vi "Cylindrical E-Field Meter.vi"() -> ()   [LabVIEW 2012]
panel:
  out "x/y":dbl
  out "ADC Reading":i64
  out "Voltage on Op Amp output":dbl
  in  "Buffering size":i32=100
  out "Continuous Measurements":dbl[](graph)
  out "N of Iterations":i32
  in  "Buffering size":i32=100
  in  "stop":bool
  in  "Ey Field (V)":dbl(knob) scale=-16000.0..16000.0
  in  "Ex Field (V)":dbl(knob) scale=-1000.0..1000.0
  out "Measurements taken every 2*Pi":dbl[](graph)
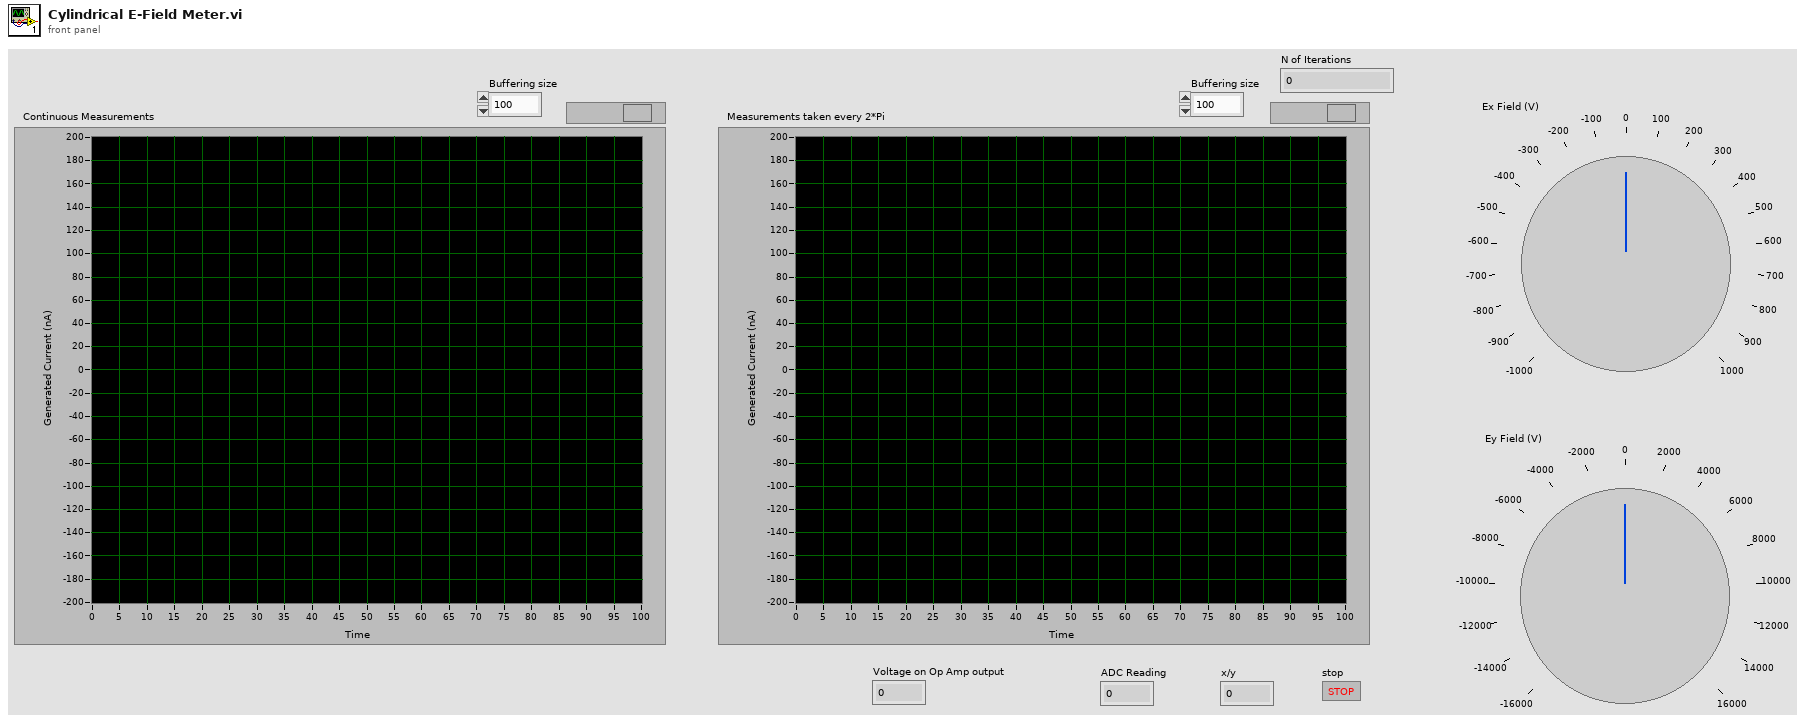
[diagram p1: front panel]
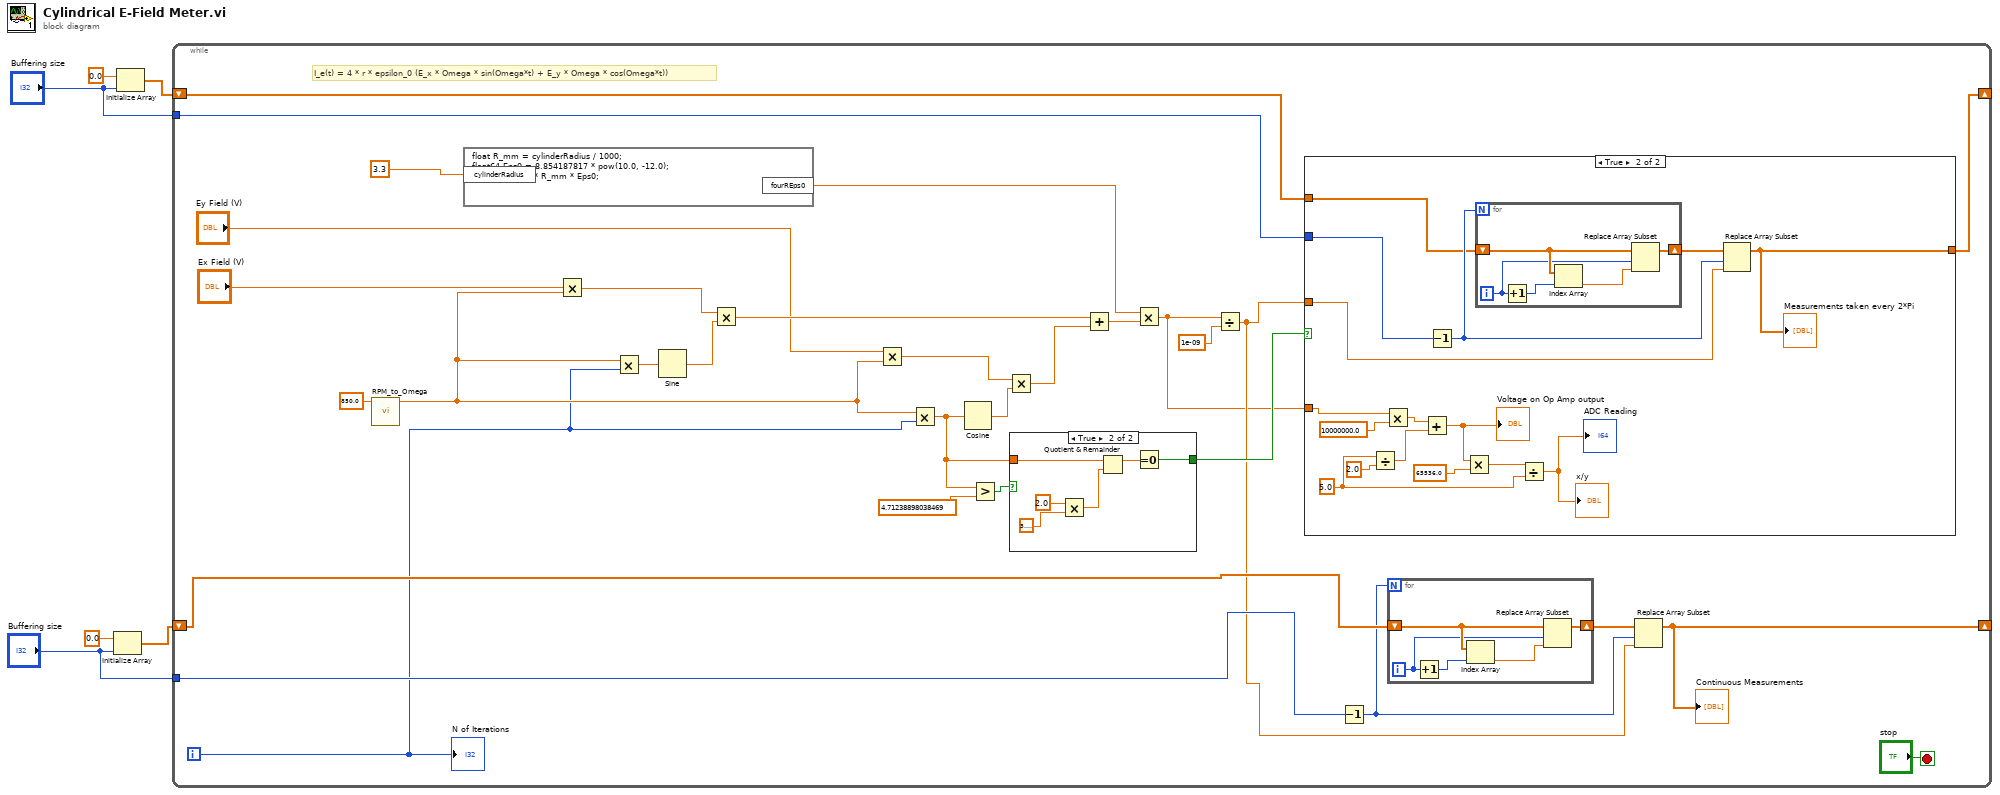
[diagram p0: block diagram]
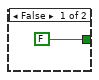
[diagram p2: hidden frame]
diagram:
  n1 = Initialize Array(0.0 ("element"), "Buffering size") -> (w3:dbl[])
  n2 = Initialize Array(0.0 ("element"), "Buffering size") -> (w5:dbl[])
  n3 = while {
    tunnel: "Buffering size" -> [w36]
    shift-right: [w34] -> _
    shift-left: w5 -> [w35]
    shift-right: [w12] -> _
    shift-left: w3 -> [w21]
    tunnel: "Buffering size" -> [w20]
    i -> [w9]
    stop <- "stop" stop-if-true
    # "I_e(t) = 4 * r * epsilon_0 (E_x * Omega * sin(Omega*t) + E_y * Omega * cos(Omega*t))"
    n4 = call "RPM_to_Omega.vi"("Rotational Speed (RPM)"=850.0) -> ("Angular Velocity (omega)"=w23:dbl)  [unwired: 10 in]
    n5 = formula code="float R_mm = cylinderRadius / 1000;\nfloat64 Eps0 = 8.854187817 * pow(10.0, -12.0);\nfourREps0 = 4 * R_mm * Eps0;"("cylinderRadius"=3.3 ("input variable")) -> ("fourREps0"=w10:dbl)
    n6 = Multiply(x="Ex Field (V)", y=w23) -> (x*y=w33:dbl)
    n7 = Multiply(x=w23, y=w9) -> (x*y=w18:dbl)
    n8 = Sine(x=w18) -> (sin(x)=w31:dbl)
    n9 = Multiply(x=w33, y=w31) -> (x*y=w29:dbl)
    n10 = Multiply(x="Ey Field (V)", y=w23) -> (x*y=w32:dbl)
    n11 = Multiply(x=w23, y=w9) -> (x*y=w16:dbl)
    n12 = Cosine(x=w16) -> (cos(x)=w30:dbl)
    n13 = Greater?(x=w16, y=4.71238898038469) -> (0:w15:bool)
    n14 = Multiply(x=w32, y=w30) -> (x*y=w28:dbl)
    n15 = case shown="True" w15 {
      tunnel: [FALSE w48] -> w22
      tunnel: w16 -> [_ w44]
      frame False {
      }
      frame True {
        n16 = Multiply(x=2.0, y=3.141592653589793) -> (x*y=w45:dbl)
        n17 = Quotient & Remainder(x=w44, y=w45) -> (x-y*floor(x/y)=w49:dbl)  [unwired: 1 out]
        n18 = Equal To 0?(x=w49) -> (x = 0?=w48:bool)
      }
    }
    n19 = Add(x=w29, y=w28) -> (x+y=w27:dbl)
    n20 = Multiply(x=w10, y=w27) -> (x*y=w11:dbl)
    n21 = Divide(x=w11, y=1e-09) -> (x/y=w19:dbl)
    n22 = case shown="True" w22 {
      tunnel: w19 -> [_ w64]
      tunnel: w36 -> [_ w63]
      tunnel: w35 -> [w50 w62]
      tunnel: [w50 w61] -> w34
      tunnel: w11 -> [_ w60]
      frame False {
      }
      frame True {
        w52 = 5.0 ("y")
        n23 = Divide(x=w52, y=2.0) -> (x/y=w51:dbl)
        n24 = Multiply(x=w60, y=10000000.0) -> (x*y=w59:dbl)
        n25 = Add(x=w59, y=w51) -> (x+y=w55:dbl)
        "Voltage on Op Amp output" <- w55
        n26 = Decrement(x=w63) -> (x-1=w65:i32)
        n27 = Multiply(x=w55, y=65536.0) -> (x*y=w57:dbl)
        n28 = for {
          N: w65 -> [_]
          shift-right: [w71] -> w66
          shift-left: w62 -> [w69]
          i -> [w67]
          n29 = Increment(x=w67) -> (x+1=w68:i32)
          n30 = Index Array(array=w69, index=w68) -> (element=w70:dbl)
          n31 = Replace Array Subset(array=w69, new element=w70, index=w67) -> (w71:dbl[])
        }
        n32 = Divide(x=w57, y=w52) -> (x/y=→"ADC Reading" →"x/y":dbl)
        n33 = Replace Array Subset(array=w66, new element=w64, index=w65) -> (w61:dbl[])
        "Measurements taken every 2*Pi" <- w61
      }
    }
    n34 = Decrement(x=w20) -> (x-1=w13:i32)
    n35 = for {
      N: w13 -> [_]
      shift-right: [w42] -> w14
      shift-left: w21 -> [w40]
      i -> [w38]
      n36 = Increment(x=w38) -> (x+1=w39:i32)
      n37 = Index Array(array=w40, index=w39) -> (element=w41:dbl)
      n38 = Replace Array Subset(array=w40, new element=w41, index=w38) -> (w42:dbl[])
    }
    n39 = Replace Array Subset(array=w14, new element=w19, index=w13) -> (w12:dbl[])
    "Continuous Measurements" <- w12
    "N of Iterations" <- w9
  }
